vi "test_Format Time (Good Time).vi"(8 "error in (no error)":errorcluster, 11 "TestCase in":refnum<class "Test-Layout.lvclass">=refnum) -> (0 "error out":errorcluster, 3 "TestCase out":refnum<class "Test-Layout.lvclass">)   [LabVIEW 2019, in "Test-Layout.lvclass"]
uses:
  Test-Layout.lvclass
  Layouts/Layout.lvclass
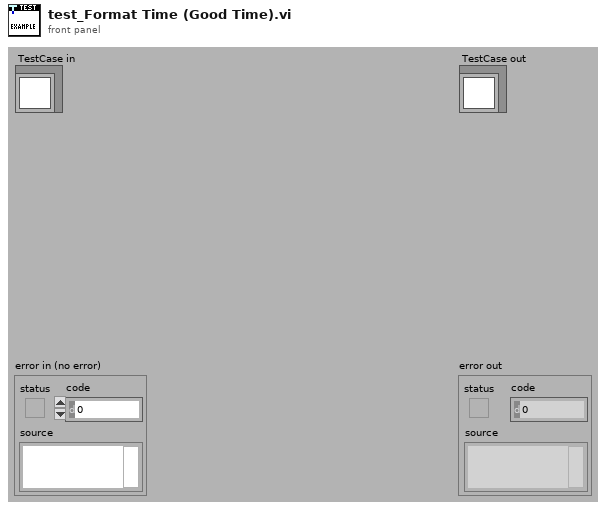
[diagram p1: front panel]
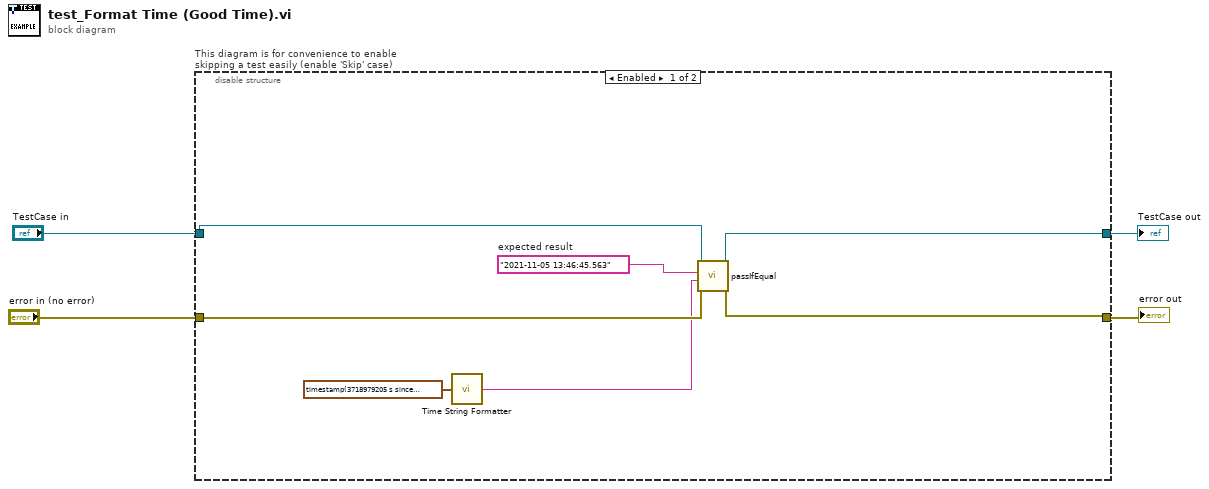
[diagram p0: block diagram]
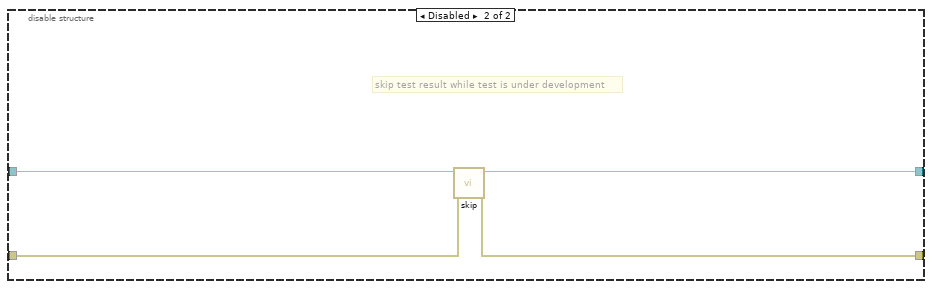
[diagram p2: hidden frame]
diagram:
  n1 = disable-structure "This diagram is for convenience to enable skipping a test easily (enable 'Skip' case)" shown="Enabled" {
    disable-tunnel: "TestCase in" -> [w10 w15]
    disable-tunnel: [w9 w13] -> w1
    disable-tunnel: [w8 w14] -> w3
    disable-tunnel: "error in (no error)" -> [w7 w12]
    frame Enabled {
      w11 = "2021-11-05 13:46:45.563"  # expected result
      n2 = call "Time String Formatter.vi"("Time"=timestamp(3718979205.5636735 s since 1904-01-01)) -> ("Time string"=w6:string)
      n3 = call-dynamic "passIfEqual.vi"("error in (no error)"=w7, "y"=w6, "x"=w11, "TestCase in"=w10) -> ("error out"=w8:errorcluster, "TestCase out"=w9:refnum<class "Test-Layout.lvclass">)  [unwired: 6 in]
    }
    frame Disabled {
      # "skip test result while test is under development"
      n4 = call <vilib>:"skip.vi"("error in (no error)"=w12, "TestCase in"=w15) -> ("error out"=w14:errorcluster, "TestCase out"=w13:refnum<class "Test-Layout.lvclass">)  [unwired: 8 in]
    }
  }
  "error out" <- w3
  "TestCase out" <- w1
